vi "IFD Strip Offset Fill.vi"(8 "error in (no error)":errorcluster, 10 "refnum":refnum<file>, 11 "IFD in":refnum<class "IFD.lvclass">) -> (0 "error out":errorcluster, 2 "refnum out":refnum<file>, 3 "IFD out":refnum<class "IFD.lvclass">)   [LabVIEW 2016, in "IFD.lvclass"]
uses:
  IFD.lvclass
  IFD.lvclass/IFD.ctl
  Tag/IFD_Tag.lvclass/IFD_Tag.ctl
  Tag/Tag Size.vi
  Tag/IFD_Tag.lvclass
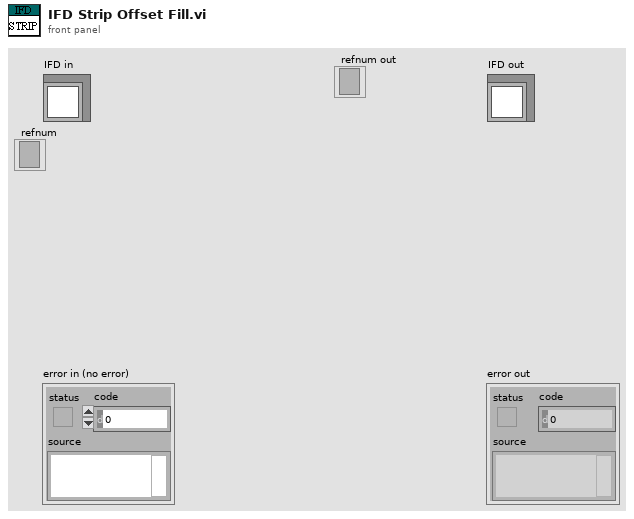
[diagram p1: front panel]
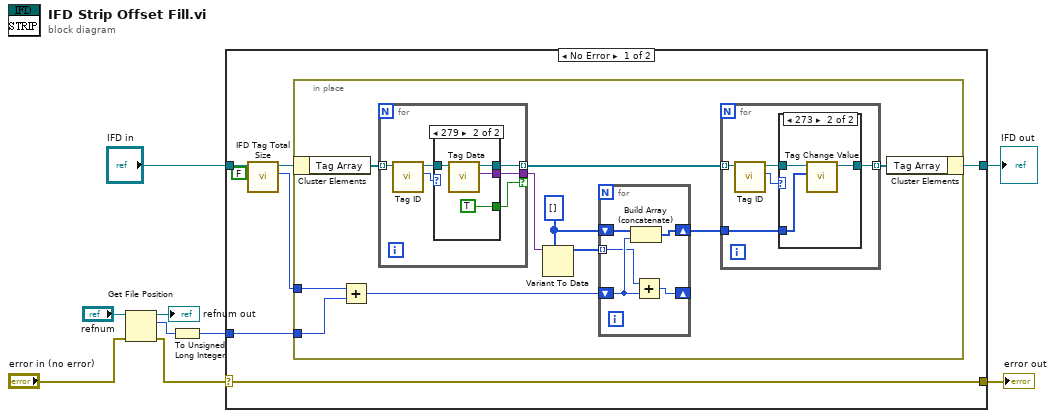
[diagram p0: block diagram]
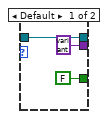
[diagram p3: hidden frame]
diagram:
  n1 = Get File Position(4:"error in (no error)", 7:"refnum") -> (0:w1:errorcluster, 2:w4:i64, 3:→"refnum out":refnum<file>)
  n2 = To Unsigned Long Integer(number=w4) -> (unsigned 32bit integer=w3:u32)
  n3 = case shown="No Error" w1 {
    selector: w1 -> [w16 w55]
    tunnel: [w16 w55] -> w9
    tunnel: [w13 w54] -> w7
    tunnel: "IFD in" -> [w15 w54]
    tunnel: w3 -> [w11 _]
    frame No Error {
      n4 = call "IFD Tag Total Size.vi"("Add Strip"=FALSE, "IFD in"=w15) -> ("Size(byte)"=w12:u32, "IFD out"=w14:refnum<class "IFD.lvclass">)  [unwired: 7 in, 1 out]
      n5 = in-place {
        in-place-border: w12 -> [w24]
        in-place-border: w11 -> [w23]
        w18 = u32[] []
        n6 = in-place-cluster #1(w14) -> ("Tag Array"=w26:refnum<class "IFD_Tag.lvclass">[])
        n7 = Add(x=w24, y=w23) -> (x+y=w21:u32)
        n8 = for {
          tunnel: w26 -> [w46] mode=indexing
          tunnel: [w43] -> w22 mode=indexing
          tunnel: [w42] -> w25 if=w41
          n9 = call "Tag ID.vi"("IFD_Tag in"=w46) -> ("Tag ID"=w45:u16, "IFD_Tag out"=w44:refnum<class "IFD_Tag.lvclass">)  [unwired: 8 in, 1 out]
          n10 = case shown="279" w45 {
            tunnel: w44 -> [w49 w53]
            tunnel: [w49 w52] -> w43
            tunnel: [variant ("Data(Varient)") w51] -> w42
            tunnel: [FALSE TRUE] -> w41
            frame Default {
            }
            frame 279 {
              n11 = call "Tag Data.vi"("IFD_Tag in"=w53) -> ("Data(Varient)"=w51:variant, "IFD_Tag out"=w52:refnum<class "IFD_Tag.lvclass">)  [unwired: 8 in, 1 out]
            }
          }
        }
        n12 = Variant To Data(type=w18, Variant=w25) -> (data=w20:u32[])  [unwired: 1 in, 1 out]
        n13 = for {
          tunnel: w20 -> [w28] mode=indexing
          shift-right: [w30] -> w17
          shift-left: w18 -> [w31]
          shift-right: [w27] -> _
          shift-left: w21 -> [w29]
          n14 = Build Array (concatenate)(w31, w29) -> (w30:u32[])
          n15 = Add(x=w28, y=w29) -> (x+y=w27:u32)
        }
        n16 = for {
          tunnel: w22 -> [w36] mode=indexing
          tunnel: [w33] -> w19 mode=indexing
          tunnel: w17 -> [w32]
          n17 = call "Tag ID.vi"("IFD_Tag in"=w36) -> ("Tag ID"=w35:u16, "IFD_Tag out"=w34:refnum<class "IFD_Tag.lvclass">)  [unwired: 8 in, 1 out]
          n18 = case shown="273" w35 {
            tunnel: w34 -> [w37 w40]
            tunnel: [w37 w38] -> w33
            tunnel: w32 -> [_ w39]
            frame Default {
            }
            frame 273 {
              n19 = call "Tag Change Value.vi"("Data"=w39, "IFD_Tag in"=w40) -> ("IFD_Tag out"=w38:refnum<class "IFD_Tag.lvclass">)  [unwired: 9 in]
            }
          }
        }
        n20 = in-place-cluster #1("Tag Array"=w19) -> (w13:refnum<class "IFD.lvclass">)
      }
    }
    frame Error {
    }
  }
  "error out" <- w9
  "IFD out" <- w7
